vi "testPassed.vi"() -> (0 "error out":errorcluster)   [LabVIEW 2019, in "TestResultTest.lvlib"]
uses:
  TestResultTest.lvlib
  TestResult/TestResult.lvclass
  Support/TestCaseMock/TestCaseMock.lvclass
  C:/Users/de200256/Code/LVUnit/TestCase/TestCase/TestCase.lvclass
  Assertion/Assertion.lvlib
  C:/Users/de200256/Code/LVUnit/Test/Test.lvclass
  TestCase/TestCase/TestCase.lvclass
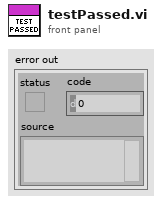
[diagram p1: front panel]
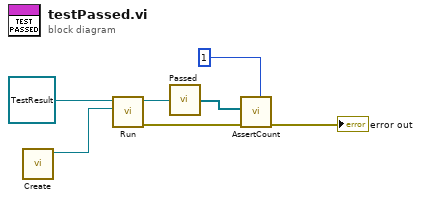
[diagram p0: block diagram]
diagram:
  n1 = call "Create.vi"() -> ("TestCaseMock"=w1:refnum<class "TestCaseMock.lvclass">)  [unwired: 10 in, 1 out]
  n2 = call-dynamic "Run.vi"("TestCase"=w1, "TestResult in"=refnum<class "TestResult.lvclass"> refnum ("TestResult.lvclass")) -> ("error out"=w4:errorcluster, "TestResult out"=w6:refnum<class "TestResult.lvclass">)  [unwired: 7 in, 1 out]
  n3 = call "Passed.vi"("TestResult In"=w6) -> ("Passed"=w5:refnum<class "TestCase.lvclass">[])
  n4 = call "AssertCount.vi"("Expected"=1, "error in (no error)"=w4, "Haystack"=w5) -> ("error out"=→"error out":errorcluster)  [unwired: 8 in]
